vi "FRCts20_EspEngine_ConvertToUniverse.vi"(8 "error in (no error)":errorcluster, 9 "Events":T11, 10 "Teams":T10) -> (0 "error out":errorcluster, 2 "Universe":T1)   [LabVIEW 2014, in "FRCts20_EspEngine.lvlib"]
uses:
  FRCts20_EspEngine.lvlib
  Web Methods/source/VI Source/Web Method Public Interface/FRCts20_WebMethods_ctl_events.ctl
  Web Methods/source/VI Source/Web Method Public Interface/FRCts20_WebMethods_ctl_teamIdentifier.ctl
  Web Methods/source/VI Source/Web Method Public Interface/FRCts20_WebMethods_ctl_singleEvent.ctl
  Web Methods/source/VI Source/Web Method Public Interface/FRCts20_WebMethods_ctl_teams.ctl
  Web Methods/source/VI Source/Web Method Public Interface/FRCts20_WebMethods_ctl_singleTeam.ctl
  Backend/source/VI Source/FRCts20_Backend_API/FRCts20_Backend_API_SW.ctl
  TypeDefs/FRCts20_EspEngine_Universe.ctl
  TypeDefs/FRCts20_EspEngine_Team.ctl
  Web Methods/source/VI Source/Web Method Public Interface/FRCts20_WebMethods_ctl_request.ctl
  Backend/source/VI Source/FRCts20_Backend_API/FRCts20_Backend_API_Status.ctl
  TypeDefs/FRCts20_EspEngine_Event.ctl
  Web Methods/source/VI Source/FRCts20_WebMethods.lvlib
  Backend/source/VI Source/FRCts20_Backend_API/FRCts20_Backend_API.lvlib
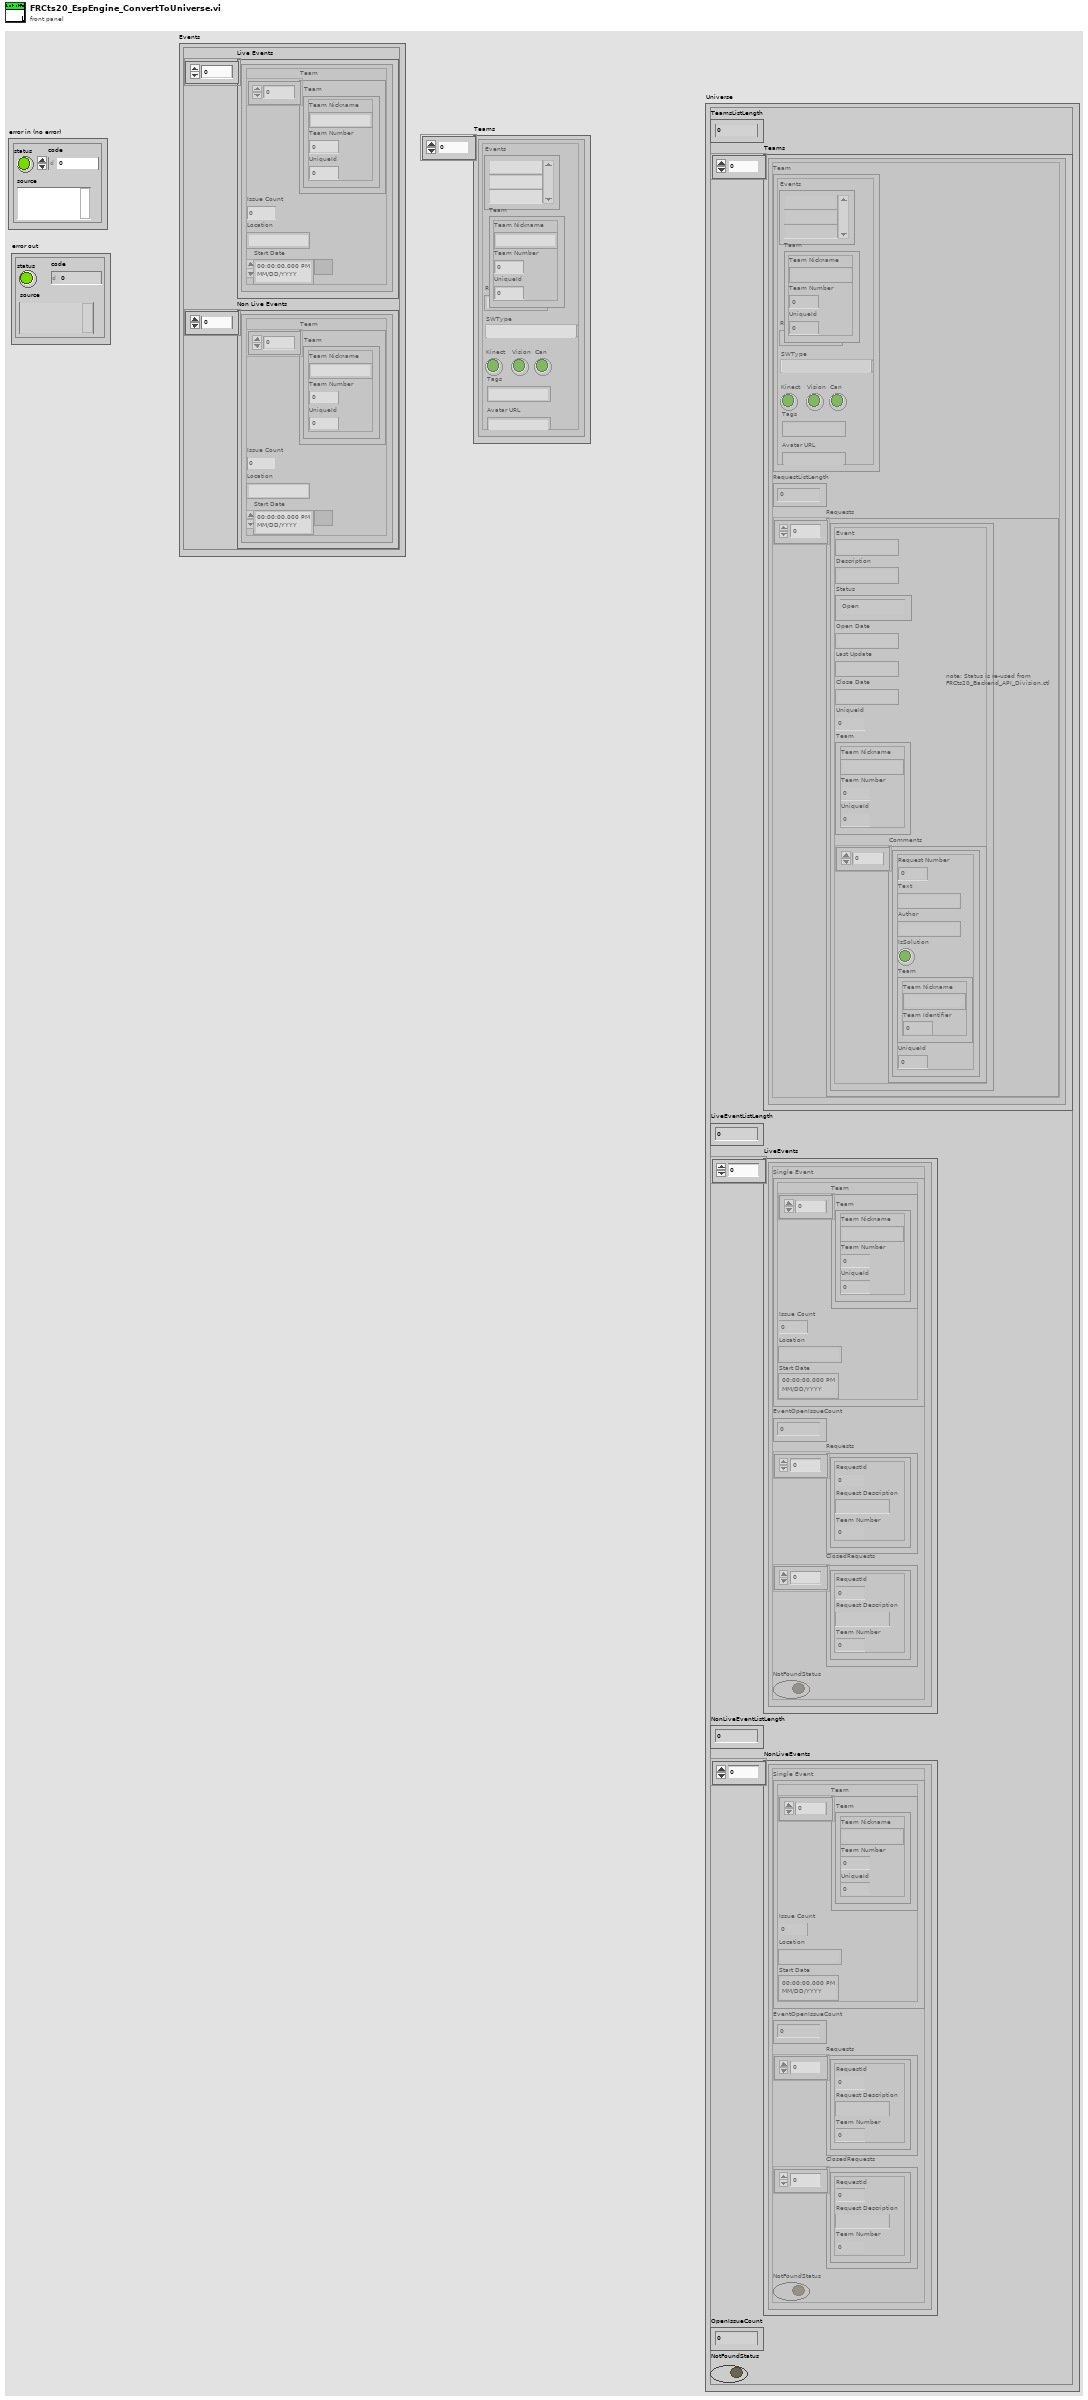
[diagram p1: front panel]
types:
  T1 = typedef "FRCts20_EspEngine.lvlib/FRCts20_EspEngine_Universe.ctl" = cluster{"TeamsListLength":i16, "Teams":T2[], "LiveEventListLength":i16, "LiveEvents":T8[], "NonLiveEventListLength":i16, "NonLiveEvents":T8[], "OpenIssueCount":i16, "NotFoundStatus":bool}
  T2 = typedef "FRCts20_EspEngine.lvlib/FRCts20_EspEngine_Team.ctl" = cluster{"Team":T3, "RequestListLength":i16, "Requests":T6[]}
  T3 = typedef "FRCts20_WebMethods.lvlib/FRCts20_WebMethods_ctl_singleTeam.ctl" = cluster{"Events":string[], "Robot Name":string, "Kinect":bool, "Vision":bool, "Can":bool, "Tags":string, "Avatar URL":string, "Team":T4, "SWType":T5}
  T4 = typedef "FRCts20_WebMethods.lvlib/FRCts20_WebMethods_ctl_teamIdentifier.ctl" = cluster{"Team Nickname":string, "Team Number ":u32, "UniqueId":u32}
  T5 = typedef "FRCts20_Backend_API.lvlib/FRCts20_Backend_API_SW.ctl" = string
  T6 = typedef "FRCts20_WebMethods.lvlib/FRCts20_WebMethods_ctl_request.ctl" = cluster{"Event":string, "Description":string, "Status":T7, "Open Date":string, "Last Update":string, "Close Date":string, "UniqueId":i32, "Team":cluster{"Team Nickname":string, "Team Number ":i32, "UniqueId":i32}, "Comments":cluster{"Request Number":dbl, "Text":string, "Author":string, "IsSolution":bool, "Team":cluster{"Team Nickname":string, "Team Identifier ":dbl}, "UniqueId":i32}[]}
  T7 = typedef "FRCts20_Backend_API.lvlib/FRCts20_Backend_API_Status.ctl" = enum16{"Open", "In Work", "Closed"}
  T8 = typedef "FRCts20_EspEngine.lvlib/FRCts20_EspEngine_Event.ctl" = cluster{"Single Event":T9, "EventOpenIssueCount":i16, "Requests":cluster{"RequestId":i32, "Request Description":string, "Team Number":i32}[], "ClosedRequests":cluster{"RequestId":i32, "Request Description":string, "Team Number":i32}[], "NotFoundStatus":bool}
  T9 = typedef "FRCts20_WebMethods.lvlib/FRCts20_WebMethods_ctl_singleEvent.ctl" = cluster{"Team":T4[], "Issue Count":i32, "Location":string, "Start Date ":timestamp}
  T10 = typedef "FRCts20_WebMethods.lvlib/FRCts20_WebMethods_ctl_teams.ctl" = T3[]
  T11 = typedef "FRCts20_WebMethods.lvlib/FRCts20_WebMethods_ctl_events.ctl" = cluster{"Live Events":cluster{"Team":T4[], "Issue Count":i32, "Location":string, "Start Date ":timestamp}[], "Non Live Events":T9[]}
  T12 = cluster{"Team":T4[], "Issue Count":i32, "Location":string, "Start Date ":timestamp}[]
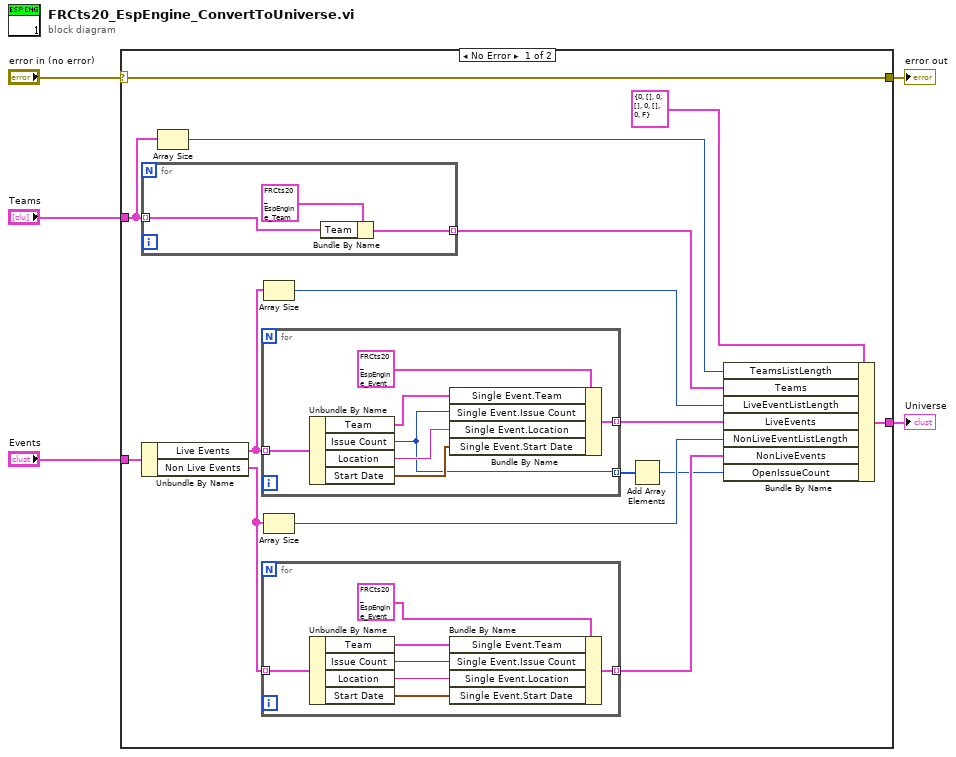
[diagram p0: block diagram]
diagram:
  n1 = case shown="No Error" "error in (no error)" {
    selector: "error in (no error)" -> [w8 w38]
    tunnel: [w8 w38] -> w5
    tunnel: "Teams" -> [w6 _]
    tunnel: "Events" -> [w19 _]
    tunnel: [w9 _] -> w1
    frame No Error {
      n2 = for {
        tunnel: w6 -> [w22] mode=indexing
        tunnel: [w21] -> w7 mode=indexing
        n3 = Bundle By Name(cluster=T2 {"Team"={"Events"=[], "Robot Name"="", "Kinect"=FALSE, "Vision"=FALSE, "Can"=FALSE, "Tags"="", "Avatar URL"="", "Team"={"Team Nickname"="", "Team Number "=0, "UniqueId"=0}, "SWType"=""}, "RequestListLength"=0, "Requests"=[]} ("Team"), "Team"=w22) -> (w21:T2)
      }
      n4 = Unbundle By Name(w19) -> ("Live Events"=w13:T12, "Non Live Events"=w15:T9[])
      n5 = Array Size(array=w6) -> (size(s)=w18:i32)
      n6 = for {
        tunnel: [w26] -> w12 mode=indexing
        tunnel: w13 -> [w25] mode=indexing
        tunnel: [w24] -> w11 mode=indexing
        n7 = Unbundle By Name(w25) -> ("Team"=w29:T4[], "Issue Count"=w24:i32, "Location"=w28:string, "Start Date"=w27:timestamp)
        n8 = Bundle By Name(cluster=T8 {"Single Event"={"Team"=[], "Issue Count"=0, "Location"="", "Start Date "=timestamp(0 s since 1904-01-01)}, "EventOpenIssueCount"=0, "Requests"=[], "ClosedRequests"=[], "NotFoundStatus"=FALSE} ("Event"), "Single Event.Team"=w29, "Single Event.Issue Count"=w24, "Single Event.Location"=w28, "Single Event.Start Date"=w27) -> (w26:T8)
      }
      n9 = for {
        tunnel: w15 -> [w37] mode=indexing
        tunnel: [w31] -> w14 mode=indexing
        n10 = Unbundle By Name(w37) -> ("Team"=w35:T4[], "Issue Count"=w34:i32, "Location"=w33:string, "Start Date"=w32:timestamp)
        n11 = Bundle By Name(cluster=T8 {"Single Event"={"Team"=[], "Issue Count"=0, "Location"="", "Start Date "=timestamp(0 s since 1904-01-01)}, "EventOpenIssueCount"=0, "Requests"=[], "ClosedRequests"=[], "NotFoundStatus"=FALSE} ("Event"), "Single Event.Team"=w35, "Single Event.Issue Count"=w34, "Single Event.Location"=w33, "Single Event.Start Date"=w32) -> (w31:T8)
      }
      n12 = Array Size(array=w13) -> (size(s)=w17:i32)
      n13 = Array Size(array=w15) -> (size(s)=w16:i32)
      n14 = Add Array Elements(numeric array=w11) -> (sum=w10:i32)
      n15 = Bundle By Name(cluster=T1 {"TeamsListLength"=0, "Teams"=[], "LiveEventListLength"=0, "LiveEvents"=[], "NonLiveEventListLength"=0, "NonLiveEvents"=[], "OpenIssueCount"=0, "NotFoundStatus"=FALSE} ("Universe"), "TeamsListLength"=w18, "Teams"=w7, "LiveEventListLength"=w17, "LiveEvents"=w12, "NonLiveEventListLength"=w16, "NonLiveEvents"=w14, "OpenIssueCount"=w10) -> (w9:T1)
    }
    frame Error {
    }
  }
  "error out" <- w5
  "Universe" <- w1
